vi "Check if configuration files exist.vi"(8 "error in (no error)":errorcluster, 11 "ImageStackBase in":refnum<class "ImageStack.lvclass">) -> (0 "error out":errorcluster, 2 "configuration file exists?":bool, 3 "ImageStackBase out":refnum<class "ImageStack.lvclass">)   [LabVIEW 2012]
doc: "Checks whether all required configuration files for the component exist."
uses:
  ImageStack.lvclass
  <vilib>/Distrio/Murmex/Murmex/Murmex.lvclass
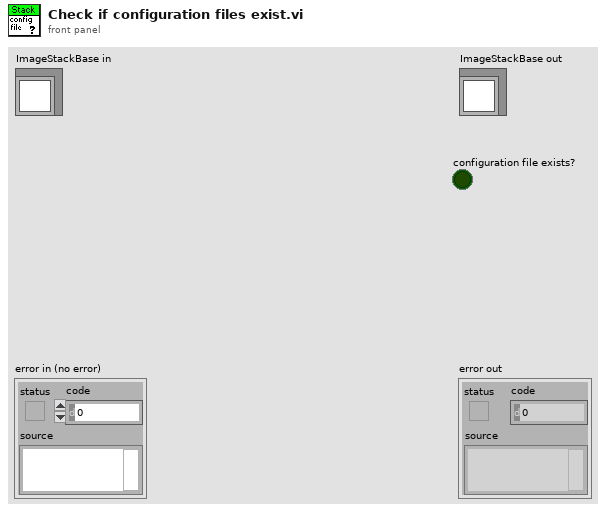
[diagram p1: front panel]
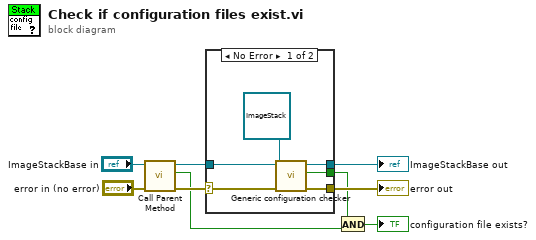
[diagram p0: block diagram]
diagram:
  n1 = call-parent "Call Parent Method"("error in (no error)"="error in (no error)", "MurmexBase in"="ImageStackBase in") -> ("error out"=w4:errorcluster, "configuration file exists?"=w2:bool, "MurmexBase out"=w7:refnum<class "ImageStack.lvclass">)  [unwired: 7 in]
  n2 = case shown="No Error" w4 {
    selector: w4 -> [w11 w16]
    tunnel: w7 -> [w15 w17]
    tunnel: [w13 w16] -> w6
    tunnel: [w12 w17] -> w5
    tunnel: [w10 _] -> w3
    frame No Error {
      n3 = call <vilib>:"Generic configuration checker.vi"("error in (no error)"=w11, 10:refnum<class "ImageStack.lvclass"> refnum ("ImageStack"), "Murmex in"=w15) -> ("error out"=w13:errorcluster, "configuration file exists?"=w10:bool, "Murmex out"=w12:refnum<class "ImageStack.lvclass">)  [unwired: 6 in]
    }
    frame Error {
    }
  }
  "error out" <- w6
  "ImageStackBase out" <- w5
  n4 = And(x=w3, y=w2) -> (x .and. y?=→"configuration file exists?":bool)
